vi "Set DataRateLevel.vi"(6 "timeout (ms)":i32=-1, 8 "error in (no error)":errorcluster, 9 "channel_name":string, 10 "Data Rate Level":T1, 11 "FlexLogger_gRPC in":refnum<class "FlexLogger_gRPC.lvclass">) -> (0 "error out":errorcluster, 3 "FlexLogger_gRPC out":refnum<class "FlexLogger_gRPC.lvclass">)   [LabVIEW 2020, in "FlexLogger_gRPC.lvlib" / "FlexLogger_gRPC.lvclass"]
uses:
  FlexLogger_gRPC.lvclass
  Controls/Flexlogger Data Rate Level Enum.ctl
  FlexLogger_client/RPC Messages/flexlogger_SetDataRateLevelRequest.ctl
  FlexLogger_client/RPC Messages/flexlogger_ElementIdentifier.ctl
  FlexLogger_gRPC.lvclass/FlexLogger_gRPC.ctl
  FlexLogger_client/FlexLogger_client.lvlib
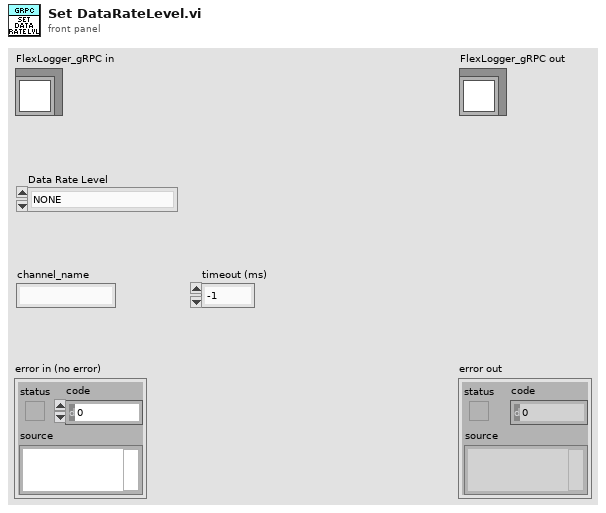
[diagram p1: front panel]
types:
  T1 = typedef "FlexLogger_gRPC.lvlib/FlexLogger_gRPC.lvclass/Flexlogger Data Rate Level Enum.ctl" = enum16{"NONE", "SLOW", "MEDIUM", "FAST", "COUNTER", "DIGITAL", "ON DEMAND"}
  T2 = typedef "FlexLogger_client.lvlib/flexlogger_SetDataRateLevelRequest.ctl" = cluster{"document_identifier":T3, "channel_name":string, "data_rate_level":i32}
  T3 = typedef "FlexLogger_client.lvlib/flexlogger_ElementIdentifier.ctl" = cluster{"project_id":string, "file_name":string, "element_id":string, "subpart_id":string}
  T4 = typedef "grpc-lvsupport-release.lvlib/grpcId.ctl" = u64
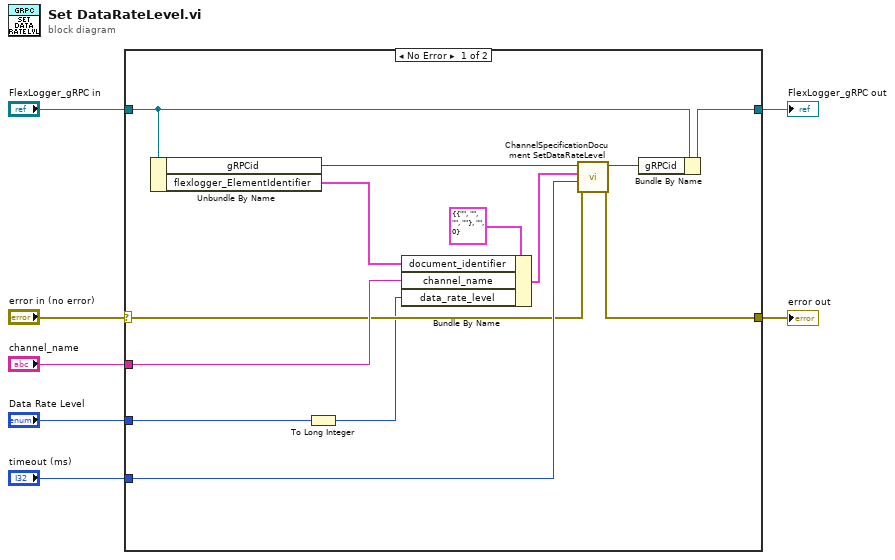
[diagram p0: block diagram]
diagram:
  n1 = case shown="No Error" "error in (no error)" {
    selector: "error in (no error)" -> [w11 w21]
    tunnel: "FlexLogger_gRPC in" -> [w20 w22]
    tunnel: [w19 w22] -> w3
    tunnel: [w14 w21] -> w4
    tunnel: "channel_name" -> [w16 _]
    tunnel: "Data Rate Level" -> [w18 _]
    tunnel: "timeout (ms)" -> [w17 _]
    frame No Error {
      n2 = Unbundle By Name(w20) -> ("gRPCid"=w13:T4, "flexlogger_ElementIdentifier"=w12:T3)
      n3 = To Long Integer(number=w18) -> (32bit integer=w8:i32)
      n4 = Bundle By Name(cluster=T2 {"document_identifier"={"project_id"="", "file_name"="", "element_id"="", "subpart_id"=""}, "channel_name"="", "data_rate_level"=0} ("Request Data"), "document_identifier"=w12, "channel_name"=w16, "data_rate_level"=w8) -> (w9:T2)
      n5 = call "ChannelSpecificationDocument SetDataRateLevel.vi"("error in"=w11, "timeout (ms)"=w17, "Request Data"=w9, "gRPC ID"=w13) -> ("error out"=w14:errorcluster, "gRPC ID out"=w15:T4)  [unwired: 5 in, 1 out]
      n6 = Bundle By Name(cluster=w20, "gRPCid"=w15) -> (w19:refnum<class "FlexLogger_gRPC.lvclass">)
    }
    frame Error {
    }
  }
  "error out" <- w4
  "FlexLogger_gRPC out" <- w3
